vi "Next Step.vi"(8 "error in (no error)":errorcluster, 11 "Magna Power Scan in":refnum<class "Magna Current Scan.lvclass">) -> (0 "error out":errorcluster, 1 "Current Step":u32, 2 "Current Position":dbl, 3 "Magna Power Scan out":refnum<class "Magna Current Scan.lvclass">)   [LabVIEW 2017, in "Magna Current Scan.lvclass"]
doc: "(Dynamic) Move to the next preconfigured step of this Scanner, and return the current position (actual, not intended) of this Scanner. Increment the step counter by one."
uses:
  Magna Current Scan.lvclass
  Scanner/Scanner.lvclass
  Instruments/Magna-Power Power Supply/Magna Power.lvclass
  C:/LabVIEW-programs-dev/Instruments/Utility Classes/Scannable/Scannable.lvclass
  C:/LabVIEW-programs-dev/Instruments/Utility Classes/Instrument/Instrument.lvclass
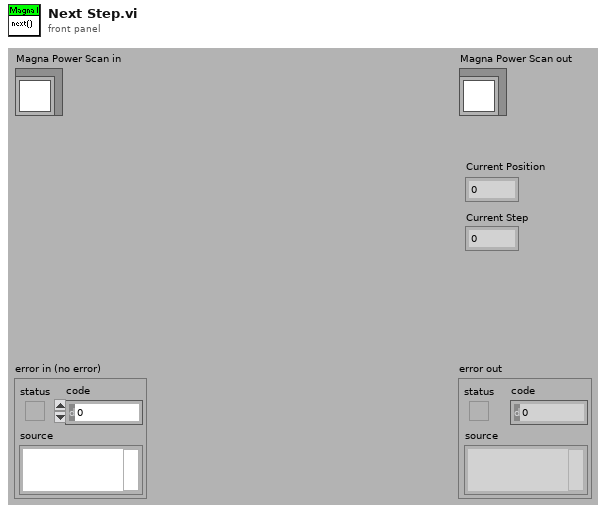
[diagram p1: front panel]
types:
  T1 = typedef "Scanner.lvclass/Range.ctl" = cluster{"xi":dbl, "xf":dbl, "dx":dbl, "Return to...?":bool, "Return to":dbl}
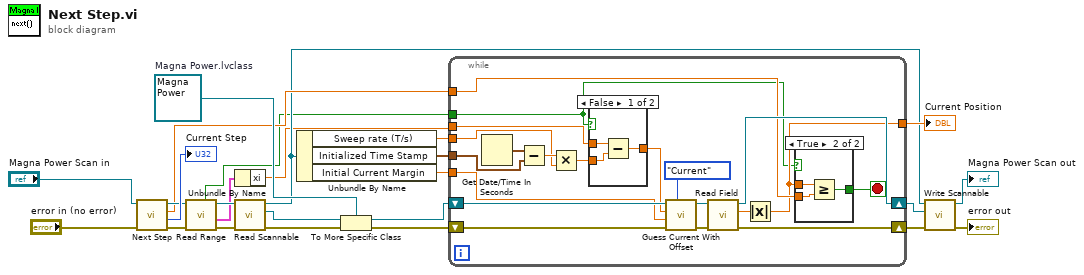
[diagram p0: block diagram]
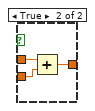
[diagram p2: hidden frame]
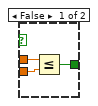
[diagram p3: hidden frame]
diagram:
  w20 = refnum<class "Magna Power.lvclass"> refnum  # Magna Power.lvclass
  n1 = call-parent "Next Step.vi"("error in (no error)"="error in (no error)", "Scanner in"="Magna Power Scan in") -> ("error out"=w19:errorcluster, "Current Step"=→"Current Step":u32, "Current Position"=w10:dbl, "Scanner out"=w17:refnum<class "Magna Current Scan.lvclass">)  [unwired: 6 in]
  n2 = call-dynamic "Read Range.vi"("error in (no error)"=w19, "Scanner.lvclass in"=w17) -> ("error out"=w18:errorcluster, "Range"=w15:T1, "Scanner.lvclass out"=w16:refnum<class "Magna Current Scan.lvclass">, "Scanning Up?"=w3:bool)  [unwired: 4 in, 2 out]
  n3 = Unbundle By Name(w15) -> ("xi"=w2:dbl)
  n4 = call-dynamic "Read Scannable.vi"("error in (no error)"=w18, "Scanner.lvclass in"=w16) -> ("error out"=w22:errorcluster, "Scannable.lvclass"=w21:refnum<class "Scannable.lvclass">, "Scanner.lvclass out"=w4:refnum<class "Magna Current Scan.lvclass">)  [unwired: 7 in]
  n5 = Unbundle By Name(w4) -> ("Sweep rate (T/s)"=w13:dbl, "Initialized Time Stamp"=w14:timestamp, "Initial Current Margin"=w1:dbl)
  n6 = To More Specific Class(target class=w20, reference=w21, error in=w22) -> (specific class reference=w11:refnum<class "Magna Power.lvclass">, error out=w12:errorcluster)
  n7 = while {
    tunnel: w14 -> [w44]
    tunnel: w13 -> [w42]
    shift-right: [w35] -> w8
    shift-left: w12 -> [w41]
    shift-right: [w36] -> w7
    shift-left: w11 -> [w40]
    tunnel: w3 -> [w30]
    tunnel: w10 -> [w34]
    tunnel: [w31] -> w9
    tunnel: w2 -> [w29]
    tunnel: w1 -> [w27]
    stop <- w33 stop-if-true
    n8 = Get Date/Time In Seconds() -> (seconds since 1Jan1904=w45:timestamp)
    n9 = Subtract(x=w45, y=w44) -> (x-y=w43:dbl)
    n10 = Multiply(x=w43, y=w42) -> (x*y=w28:dbl)
    n11 = case shown="False" w30 {
      tunnel: [w48 w51] -> w39
      tunnel: w29 -> [w47 w50]
      tunnel: w28 -> [w46 w49]
      frame False {
        n12 = Subtract(x=w47, y=w46) -> (x-y=w48:dbl)
      }
      frame True {
        n13 = Add(x=w50, y=w49) -> (x+y=w51:dbl)
      }
    }
    n14 = call "Guess Current With Offset.vi"("V or I?"=enum16{"Voltage", "Current"}."Current", "error in (no error)"=w41, "Offset"=w27, "Desired Field"=w39, "Magna Power in"=w40) -> ("error out"=w38:errorcluster, "Magna Power out"=w37:refnum<class "Magna Power.lvclass">)  [unwired: 4 in, 1 out]
    n15 = call "Read Field.vi"("error in (no error)"=w38, "Magna Power in"=w37) -> ("error out"=w35:errorcluster, "Field (T)"=w32:dbl, "Magna Power out"=w36:refnum<class "Magna Power.lvclass">)  [unwired: 5 in, 2 out]
    n16 = Absolute Value(x=w32) -> (abs(x)=w31:dbl)
    n17 = case shown="True" w30 {
      tunnel: w31 -> [w54 w55]
      tunnel: w34 -> [w53 w57]
      tunnel: [w52 w56] -> w33
      frame False {
        n18 = Less Or Equal?(x=w54, y=w53) -> (x <= y?=w52:bool)
      }
      frame True {
        n19 = Greater Or Equal?(x=w55, y=w57) -> (x >= y?=w56:bool)
      }
    }
  }
  "Current Position" <- w9
  n20 = call-dynamic "Write Scannable.vi"("error in (no error)"=w8, "Scannable.lvclass"=w7, "Scanner.lvclass in"=w4) -> ("error out"=→"error out":errorcluster, "Scanner.lvclass out"=→"Magna Power Scan out":refnum<class "Magna Current Scan.lvclass">)  [unwired: 7 in]
